vi "Get Sensor Tiles Info.vi"(8 "error in (no error)":errorcluster, 11 "Abstract Sensor Tiles Info Msg in":refnum<class "Abstract Sensor Tiles Info Msg.lvclass">) -> (0 "error out":errorcluster, 2 "Sensor Tiles Info":string[][](array[string]), 3 "Abstract Sensor Tiles Info Msg out":refnum<class "Abstract Sensor Tiles Info Msg.lvclass">)   [LabVIEW 2013, in "Sensor Model.lvlib" / "Abstract Sensor Tiles Info Msg.lvclass"]
uses:
  Abstract Sensor Tiles Info Msg.lvclass
  Abstract Sensor Tiles Info Msg.lvclass/Abstract Sensor Tiles Info Msg.ctl
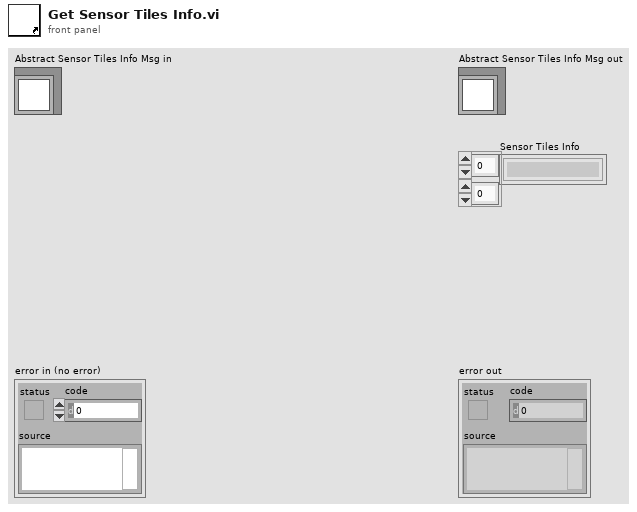
[diagram p1: front panel]
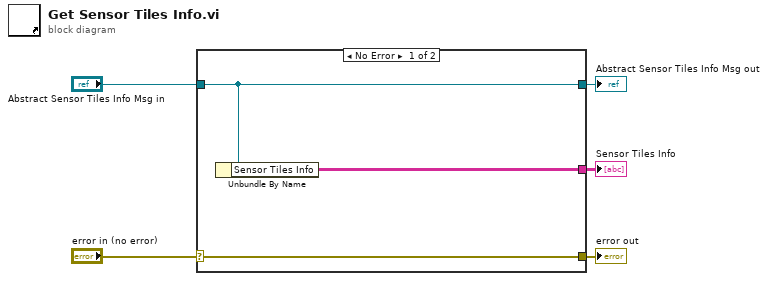
[diagram p0: block diagram]
diagram:
  n1 = case shown="No Error" "error in (no error)" {
    selector: "error in (no error)" -> [w8 w9]
    tunnel: [w8 w9] -> w4
    tunnel: [w7 w10] -> w2
    tunnel: "Abstract Sensor Tiles Info Msg in" -> [w7 w10]
    tunnel: [w6 _] -> w1
    frame No Error {
      n2 = Unbundle By Name(w7) -> ("Sensor Tiles Info"=w6:string[][])
    }
    frame Error {
    }
  }
  "error out" <- w4
  "Abstract Sensor Tiles Info Msg out" <- w2
  "Sensor Tiles Info" <- w1
